vi "Query IO.vi"(8 "error in":errorcluster, 11 "6509 in":refnum<class "6509.lvclass">) -> (0 "error out":errorcluster, 1 "Port Array":u8[](array[numeric]), 2 "Boolean Array":bool[](array[boolean]), 3 "6509 out":refnum<class "6509.lvclass">)   [LabVIEW 2019, in "6509.lvlib" / "6509.lvclass"]
doc: "This method must be overridden by the child class.\n\nThis should read the status at the output of the device and return a weform capture of the named signal states."
uses:
  Library/6509.lvclass
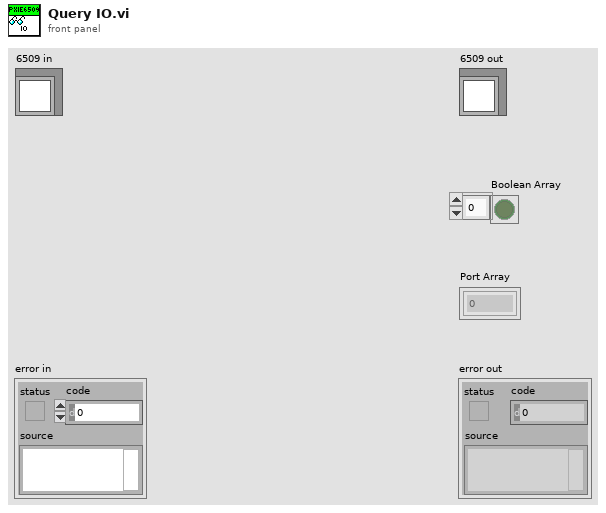
[diagram p1: front panel]
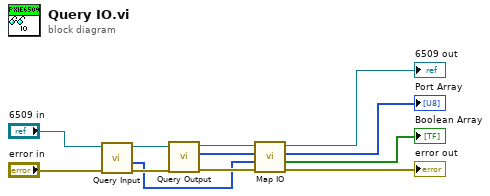
[diagram p0: block diagram]
diagram:
  n1 = call "Query Input.vi"("error in"="error in", "6509 in"="6509 in") -> ("error out"=w10:errorcluster, "Bank"=w3:u8[], "6509 out"=w11:refnum<class "6509.lvclass">)  [unwired: 7 in]
  n2 = call "Query Output.vi"("error in"=w10, "6509 in"=w11) -> ("error out"=w7:errorcluster, "Port Array"=w4:u8[], "6509 out"=w8:refnum<class "6509.lvclass">)  [unwired: 7 in]
  n3 = call "Map IO.vi"("error in (no error)"=w7, "Input Array"=w3, "Output Array"=w4, "6509 in"=w8) -> ("error out"=→"error out":errorcluster, "Boolean Array"=→"Boolean Array":bool[], "Bank Array"=→"Port Array":u8[], "6509 out"=→"6509 out":refnum<class "6509.lvclass">)  [unwired: 4 in]
